vi "PID SP Limiter.vi"(7 "SpLim_State":T2, 8 "REG param":T3={"proportional gain (Kc)"=1.0, "integral time (Ti, s)"=10.0, "derivative time (Td, s)"=1.0, "output high"=100.0, "output high start"=40.0, "output high stop"=40.0, "alr value"=0.0, "output low"=0.0, "output rate (EGU/s)"=5.0, "setpoint max"=100.0, "setpoint rate (EGU/min)"=10.0, "stop rate (EGU/min)"=5.0} {"setpoint max" format="%.2f"; "stop rate (EGU/min)" min=0.001 format="%.2f"; "setpoint rate (EGU/min)" min=0.001 format="%.2f"; "output high stop" format="%.2f"; "output high start" format="%.2f"; "output rate (EGU/s)" min=0.001 format="%.2f"; "output low" format="%.2f"; "alr value" format="%.2f"; "output high" format="%.2f"; "derivative time (Td, s)" format="%.3f"; "integral time (Ti, s)" format="%.3f"; "proportional gain (Kc)" format="%.3f"}, 10 "PV":dbl, 11 "SP":dbl) -> (0 "PID param":T1 {"dt (s)" format="%.3f"; "output rate (EGU/s)" format="%.2f"; "output low" format="%.2f"; "alr value" format="%.2f"; "output high" format="%.2f"; "derivative time (Td, s)" format="%.3f"; "integral time (Ti, s)" format="%.3f"; "proportional gain (Kc)" format="%.3f"}, 1 "End":bool, 2 "T":u32, 3 "output":dbl format="%.2f")   [LabVIEW 2019, in "control.lvlib"]
uses:
  control.lvlib
  ctl/control param.ctl
  ctl/SpLim_State.ctl
  ctl/PID param.ctl
  PID Timing Estimation.vi
panel:
  # "PID gains"
  # "output param"
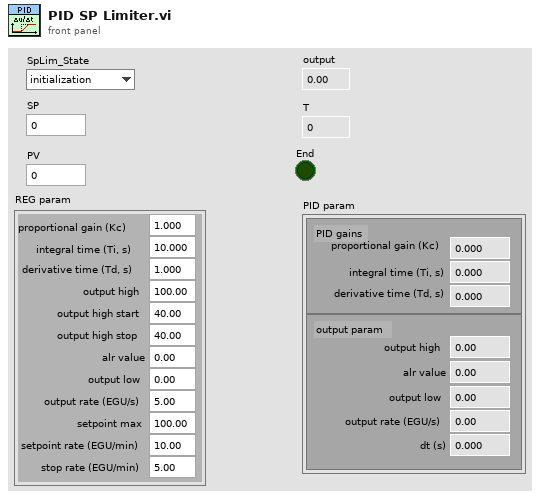
[diagram p1: front panel]
types:
  T1 = typedef "control.lvlib/PID param.ctl" = cluster{"proportional gain (Kc)":dbl, "integral time (Ti, s)":dbl, "derivative time (Td, s)":dbl, "output high":dbl, "alr value":dbl, "output low":dbl, "output rate (EGU/s)":dbl, "dt (s)":dbl}
  T2 = typedef "control.lvlib/SpLim_State.ctl" = enum8{"initialization", "stop", "decrease", "increase"}
  T3 = typedef "control.lvlib/control param.ctl" = cluster{"proportional gain (Kc)":dbl, "integral time (Ti, s)":dbl, "derivative time (Td, s)":dbl, "output high":dbl, "output high start":dbl, "output high stop":dbl, "alr value":dbl, "output low":dbl, "output rate (EGU/s)":dbl, "setpoint max":dbl, "setpoint rate (EGU/min)":dbl, "stop rate (EGU/min)":dbl}
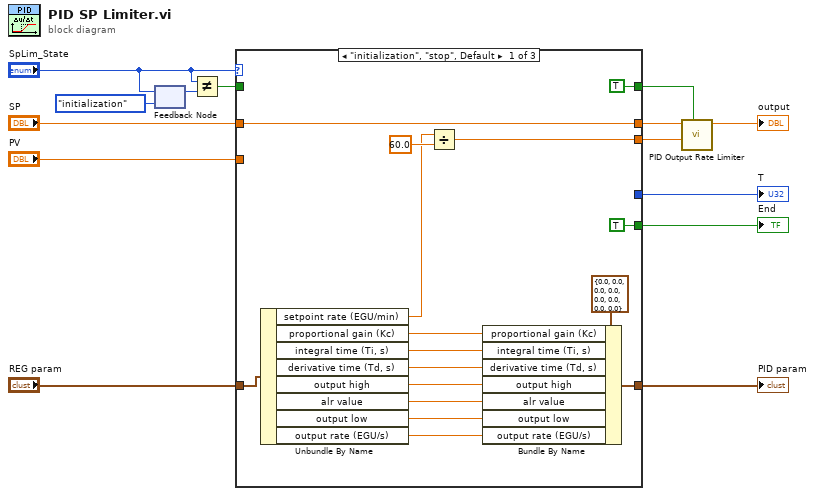
[diagram p0: block diagram]
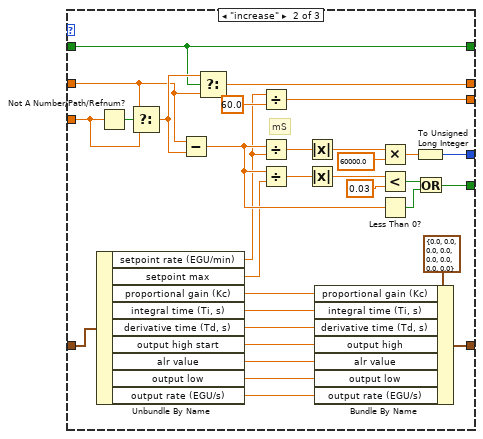
[diagram p2: hidden frame]
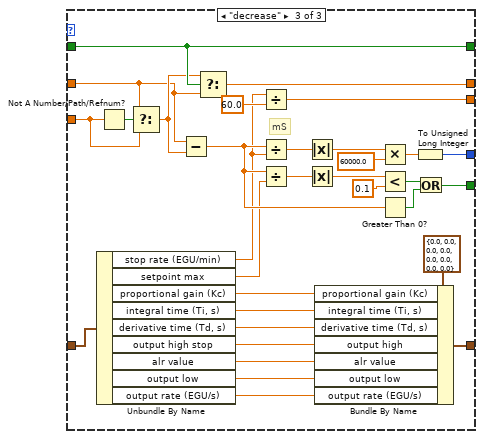
[diagram p3: hidden frame]
diagram:
  n1 = feedback #1(SpLim_State."initialization" ("SpLim_State")) -> (w7:T2)
  n2 = feedback-in #1("SpLim_State") -> ()
  n3 = Not Equal?(x="SpLim_State", y=w7) -> (x != y?=w8:bool)
  n4 = case shown="\"initialization\", \"stop\", Default" "SpLim_State" {
    tunnel: "SP" -> [w30 w37 w67]
    tunnel: "PV" -> [_ w61 w93]
    tunnel: [w30 w34 w71] -> w4
    tunnel: [_ w46 w76] -> w12
    tunnel: [TRUE w42 w74] -> w11
    tunnel: w8 -> [_ w35 w69]
    tunnel: "REG param" -> [w22 w56 w80]
    tunnel: [w21 w48 w79] -> w10
    tunnel: [w19 w36 w70] -> w3
    tunnel: [TRUE w35 w69] -> w2
    frame "initialization", "stop", Default {
      n5 = Unbundle By Name(w22) -> ("setpoint rate (EGU/min)"=w18:dbl, "proportional gain (Kc)"=w29:dbl, "integral time (Ti, s)"=w28:dbl, "derivative time (Td, s)"=w27:dbl, "output high"=w26:dbl, "alr value"=w25:dbl, "output low"=w24:dbl, "output rate (EGU/s)"=w23:dbl)
      n6 = Divide(x=w18, y=60.0 ("x")) -> (x/y=w19:dbl)
      n7 = Bundle By Name(cluster=T1 {"proportional gain (Kc)"=0.0, "integral time (Ti, s)"=0.0, "derivative time (Td, s)"=0.0, "output high"=0.0, "alr value"=0.0, "output low"=0.0, "output rate (EGU/s)"=0.0, "dt (s)"=0.0} ("PID param"), "proportional gain (Kc)"=w29, "integral time (Ti, s)"=w28, "derivative time (Td, s)"=w27, "output high"=w26, "alr value"=w25, "output low"=w24, "output rate (EGU/s)"=w23) -> (w21:T1)
    }
    frame "increase" {
      # "mS"
      n8 = Unbundle By Name(w56) -> ("setpoint rate (EGU/min)"=w33:dbl, "setpoint max"=w32:dbl, "proportional gain (Kc)"=w55:dbl, "integral time (Ti, s)"=w54:dbl, "derivative time (Td, s)"=w53:dbl, "output high start"=w52:dbl, "alr value"=w51:dbl, "output low"=w50:dbl, "output rate (EGU/s)"=w49:dbl)
      n9 = Not A Number/Path/Refnum?(number/path/refnum=w61) -> (NaN/Path/Refnum?=w62:bool)
      n10 = Select(t=w37, s=w62, f=w61) -> (s? t:f=w39:dbl)
      n11 = Subtract(x=w37, y=w39) -> (x-y=w43:dbl)
      n12 = Select(t=w39, s=w35, f=w37) -> (s? t:f=w34:dbl)
      n13 = Divide(x=w33, y=60.0 ("x")) -> (x/y=w36:dbl)
      n14 = Divide(x=w43, y=w33) -> (x/y=w59:dbl)
      n15 = Divide(x=w43, y=w32) -> (x/y=w58:dbl)
      n16 = Absolute Value(x=w59) -> (abs(x)=w45:dbl)
      n17 = Absolute Value(x=w58) -> (abs(x)=w57:dbl)
      n18 = Bundle By Name(cluster=T1 {"proportional gain (Kc)"=0.0, "integral time (Ti, s)"=0.0, "derivative time (Td, s)"=0.0, "output high"=0.0, "alr value"=0.0, "output low"=0.0, "output rate (EGU/s)"=0.0, "dt (s)"=0.0} ("PID param"), "proportional gain (Kc)"=w55, "integral time (Ti, s)"=w54, "derivative time (Td, s)"=w53, "output high"=w52, "alr value"=w51, "output low"=w50, "output rate (EGU/s)"=w49) -> (w48:T1)
      n19 = Multiply(x=w45, y=60000.0) -> (x*y=w47:dbl)
      n20 = Less?(x=w57, y=0.03) -> (x < y?=w41:bool)
      n21 = Less Than 0?(x=w43) -> (x < 0?=w40:bool)
      n22 = To Unsigned Long Integer(number=w47) -> (unsigned 32bit integer=w46:u32)
      n23 = Or(x=w41, y=w40) -> (x .or. y?=w42:bool)
    }
    frame "decrease" {
      # "mS"
      n24 = Unbundle By Name(w80) -> ("stop rate (EGU/min)"=w65:dbl, "setpoint max"=w64:dbl, "proportional gain (Kc)"=w87:dbl, "integral time (Ti, s)"=w86:dbl, "derivative time (Td, s)"=w85:dbl, "output high stop"=w84:dbl, "alr value"=w83:dbl, "output low"=w82:dbl, "output rate (EGU/s)"=w81:dbl)
      n25 = Not A Number/Path/Refnum?(number/path/refnum=w93) -> (NaN/Path/Refnum?=w94:bool)
      n26 = Select(t=w67, s=w94, f=w93) -> (s? t:f=w68:dbl)
      n27 = Subtract(x=w67, y=w68) -> (x-y=w66:dbl)
      n28 = Select(t=w68, s=w69, f=w67) -> (s? t:f=w71:dbl)
      n29 = Divide(x=w65, y=60.0 ("x")) -> (x/y=w70:dbl)
      n30 = Divide(x=w66, y=w65) -> (x/y=w91:dbl)
      n31 = Divide(x=w66, y=w64) -> (x/y=w90:dbl)
      n32 = Absolute Value(x=w91) -> (abs(x)=w78:dbl)
      n33 = Absolute Value(x=w90) -> (abs(x)=w89:dbl)
      n34 = Bundle By Name(cluster=T1 {"proportional gain (Kc)"=0.0, "integral time (Ti, s)"=0.0, "derivative time (Td, s)"=0.0, "output high"=0.0, "alr value"=0.0, "output low"=0.0, "output rate (EGU/s)"=0.0, "dt (s)"=0.0} ("PID param"), "proportional gain (Kc)"=w87, "integral time (Ti, s)"=w86, "derivative time (Td, s)"=w85, "output high"=w84, "alr value"=w83, "output low"=w82, "output rate (EGU/s)"=w81) -> (w79:T1)
      n35 = Multiply(x=w78, y=60000.0) -> (x*y=w77:dbl)
      n36 = Less?(x=w89, y=0.1) -> (x < y?=w88:bool)
      n37 = Greater Than 0?(x=w66) -> (x > 0?=w73:bool)
      n38 = To Unsigned Long Integer(number=w77) -> (unsigned 32bit integer=w76:u32)
      n39 = Or(x=w88, y=w73) -> (x .or. y?=w74:bool)
    }
  }
  "PID param" <- w10
  "T" <- w12
  "End" <- w11
  n40 = call "PID Output Rate Limiter.vi"("reinitialize? (F)"=w2, "output rate (EGU/s)"=w3, "input (controller output)"=w4) -> ("output"=→"output":dbl)  [unwired: 7 in, 1 out]
